vi "Example for Dropdown.vi"() -> ()   [LabVIEW 2013]
panel:
  in  "Table Control":string[][](table)
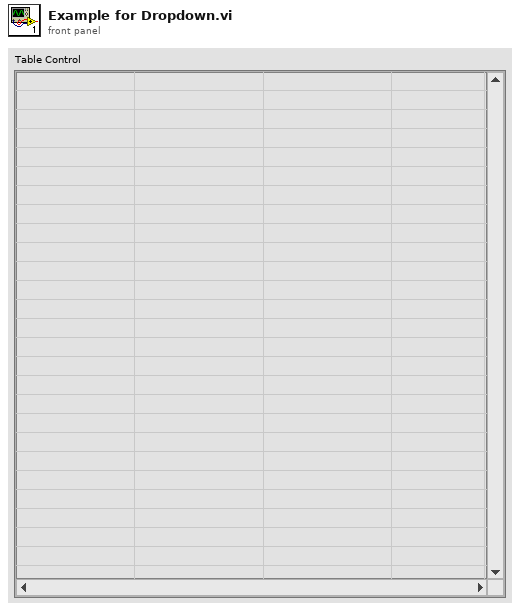
[diagram p1: front panel]
types:
  T1 = typedef "LVRowAndColumnTypeDef.ctl" = cluster{"Row":i32, "Column":i32}
  T2 = cluster{"Window Tracker":bool[], "Dropdown Visible":bool, "ActiveCell":T1}
  T3 = typedef "LVRectTypeDef.ctl" = cluster{"Left":i16, "Top":i16, "Right":i16, "Bottom":i16}
  T4 = cluster{"Table Control":refnum<vi>, "Units":string[], "Dropdown Bundle":cluster{"Window Tracker":bool[], "Dropdown Visible":bool, "ActiveCell":T1}}
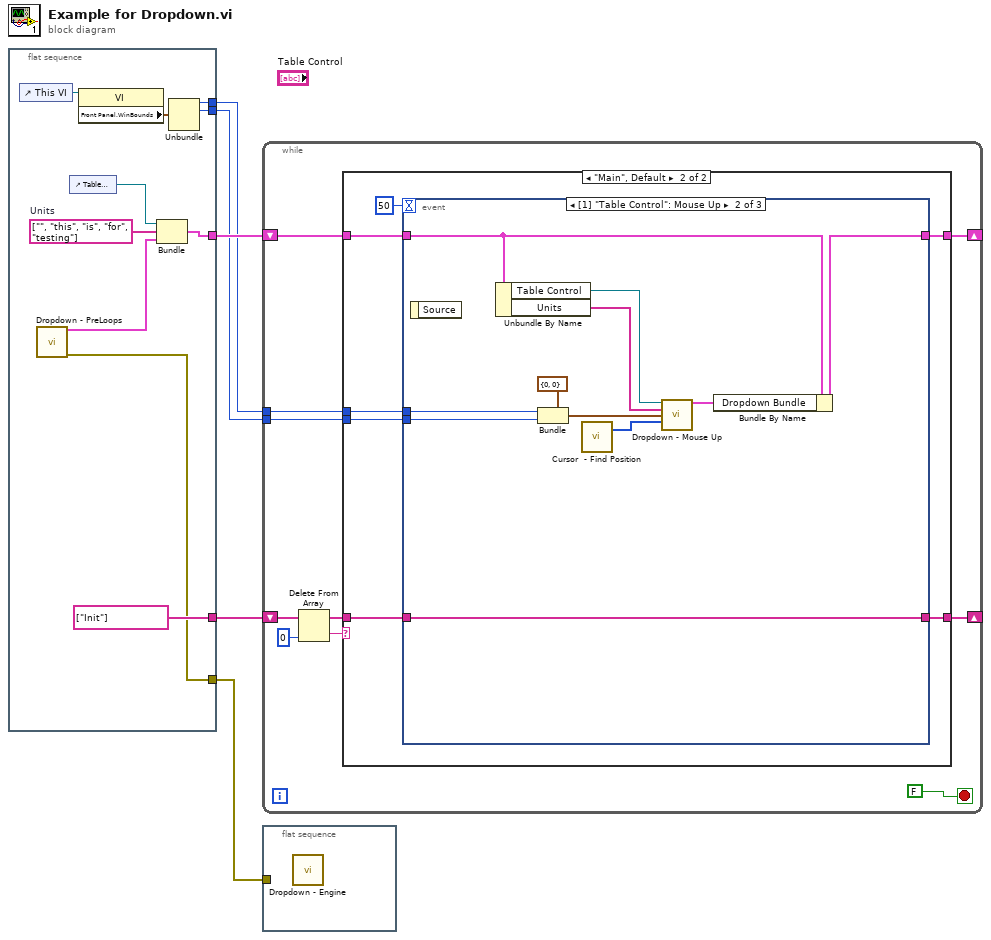
[diagram p0: block diagram]
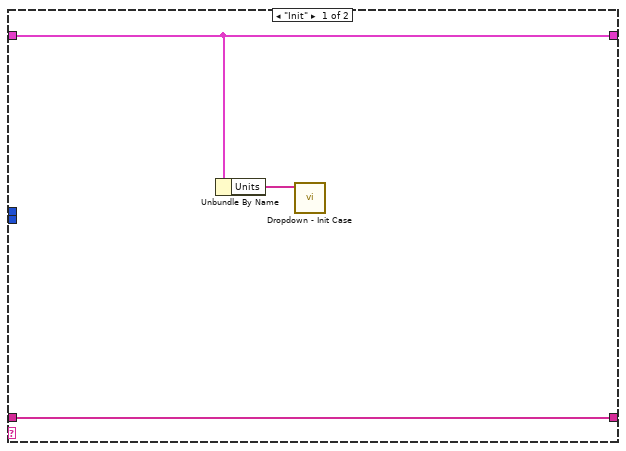
[diagram p2: hidden frame]
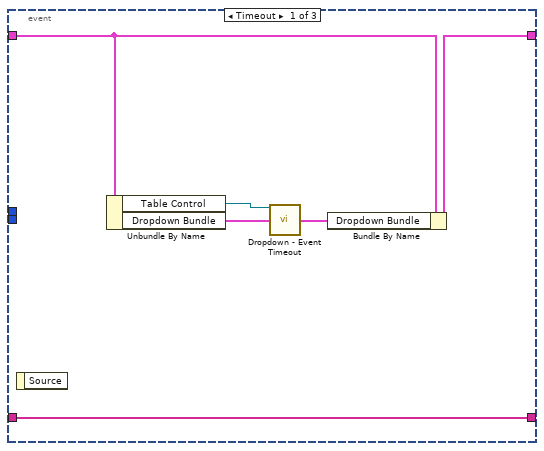
[diagram p3: hidden frame]
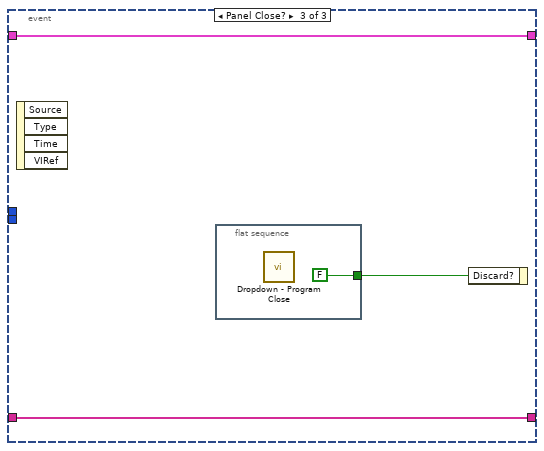
[diagram p4: hidden frame]
diagram:
  n1 = flat-sequence {
    tunnel: [w7] -> w5
    tunnel: [string[] ["Init"]] -> w4
    tunnel: [w12] -> w2
    tunnel: [w11] -> w1
    tunnel: [w10] -> w3
    frame #0 {
      w8 = string[] ["", "this", "is", "for", "testing"]  # Units
      n2 = control-ref of="This VI"() -> (w13:refnum<vi>)
      n3 = call "Dropdown - PreLoops.vi"() -> ("Dropdown Bundle"=w9:T2, "Error Out"=w10:errorcluster)  [unwired: 14 in]
      n4 = control-ref of="Table Control"() -> (w6:refnum<vi>)
      n5 = property class="VI"(reference=w13) -> ("Front Panel.WinBounds"=w14:T3)  [unwired: 1 in, 2 out]
      n6 = Bundle("Table Control"=w6, "Units"=w8, "Dropdown Bundle"=w9) -> (w7:T4)  [unwired: 1 in]
      n7 = Unbundle(w14) -> ("Left"=w12:i16, "Top"=w11:i16)  [unwired: 2 out]
    }
  }
  n8 = while {
    shift-right: [w20] -> _
    shift-left: w4 -> [w24]
    shift-right: [w18] -> _
    shift-left: w5 -> [w19]
    tunnel: w2 -> [w17]
    tunnel: w1 -> [w16]
    stop <- FALSE stop-if-true
    n9 = Delete From Array(array=w24, index=0) -> (deleted portion=w22:string, array with subset deleted=w21:string[])  [unwired: 1 in]
    n10 = case shown="\"Main\", Default" w22 {
      tunnel: w21 -> [w28 w35]
      tunnel: [w28 w33] -> w20
      tunnel: w19 -> [w27 w32]
      tunnel: [w27 w31] -> w18
      tunnel: w17 -> [_ w30]
      tunnel: w16 -> [_ w29]
      frame "Init" {
        n11 = Unbundle By Name(w27) -> ("Units"=w26:string[])
        n12 = call "Dropdown - Init Case.vi"("Unit Abbreviations"=w26) -> ()  [unwired: 10 in, 1 out]
      }
      frame "Main", Default {
        n13 = event shown="[1] \"Table Control\": Mouse Up" {
          selector: _ -> [_ _ _]
          dyn-events: _ -> [_ _ _]
          timeout: 50 -> [_ _ _]
          tunnel: w35 -> [w41 w52 w55]
          tunnel: [w41 w52 w55] -> w33
          tunnel: [w39 w43 w53] -> w31
          tunnel: w32 -> [w40 w44 w53]
          tunnel: w30 -> [_ w48 _]
          tunnel: w29 -> [_ w47 _]
          event Timeout {
            n14 = event-data() -> ()  [unwired: 1 in, 1 out]
            n15 = Unbundle By Name(w40) -> ("Table Control"=w38:refnum<vi>, "Dropdown Bundle"=w37:T2)
            n16 = call "Dropdown - Event Timeout.vi"("Table Ref"=w38, "Dropdown Bundle In"=w37) -> ("Dropdown Bundle Out"=w36:T2)  [unwired: 13 in]
            n17 = Bundle By Name(cluster=w40, "Dropdown Bundle"=w36) -> (w39:T4)
          }
          event "Table Control": Mouse Up {
            n18 = event-data() -> ()  [unwired: 1 in, 1 out]
            n19 = Unbundle By Name(w44) -> ("Table Control"=w45:refnum<vi>, "Units"=w46:string[])
            n20 = Bundle(cluster=cluster{"Left":i16, "Top":i16} {"Left"=0, "Top"=0} ("WindowPos"), "Left"=w48, "Top"=w47) -> (w49:cluster{"Left":i16, "Top":i16})
            n21 = call "Cursor  - Find Position.vi"() -> ("Cursor Position"=w51:i32[])  [unwired: 3 in]
            n22 = call "Dropdown - Mouse Up.vi"("Table Ref"=w45, "Unit Abbreviations"=w46, "WindowPos"=w49, "Cursor Position"=w51) -> ("Dropdown Bundle"=w42:T2)  [unwired: 10 in, 1 out]
            n23 = Bundle By Name(cluster=w44, "Dropdown Bundle"=w42) -> (w43:T4)
          }
          event Panel Close? {
            n24 = event-data() -> ()  [unwired: 1 in, 4 out]
            n25 = flat-sequence {
              tunnel: [FALSE] -> w54
              frame #0 {
                n26 = call "Dropdown - Program Close.vi"() -> ()  [unwired: 15 in, 1 out]
              }
            }
            n27 = event-data("Discard?"=w54) -> ()  [unwired: 1 in, 1 out]
          }
        }
      }
    }
  }
  n28 = flat-sequence {
    tunnel: w3 -> [_]
    frame #0 {
      n29 = call "Dropdown - Engine.vi"() -> ()  [unwired: 12 in]
    }
  }
